vi "Command Started.vi"(8 "error in (no error)":errorcluster, 11 "Command in":refnum<class "Command.lvclass">) -> (0 "error out":errorcluster, 3 "Command out":refnum<class "Command.lvclass">)   [LabVIEW 2013, in "Robot Actors.lvlib" / "Command.lvlib" / "Command.lvclass"]
uses:
  Command.lvclass
  Command States.ctl
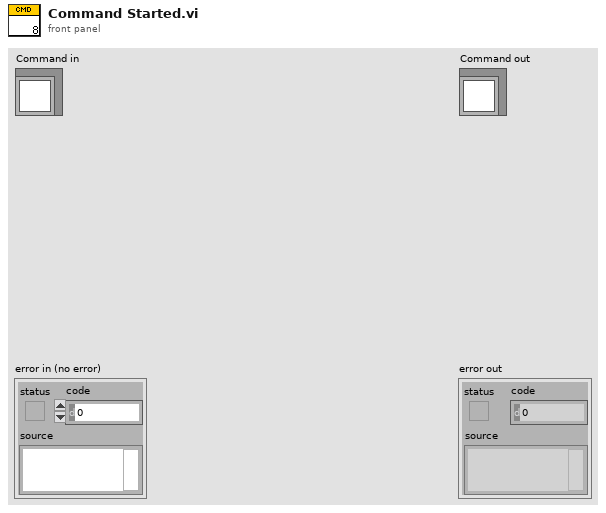
[diagram p1: front panel]
types:
  T1 = typedef "Robot Actors.lvlib/Command.lvlib/Command.lvclass/Command States.ctl" = enum16{"Unknown", "Started", "Stopped", "Finished"}
  T2 = typedef "Robot Actors.lvlib/Command.lvlib/Command.lvclass/Command Status.ctl" = cluster{"Command Name":string, "Command Start Time":timestamp, "Command End Time":timestamp, "Is Command Finished?":bool, "Command ID":dbl, "Command State":T1}
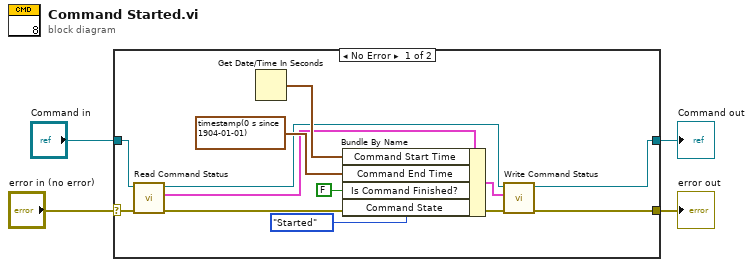
[diagram p0: block diagram]
diagram:
  n1 = case shown="No Error" "error in (no error)" {
    selector: "error in (no error)" -> [w8 w18]
    tunnel: [w6 w18] -> w3
    tunnel: [w10 w17] -> w1
    tunnel: "Command in" -> [w11 w17]
    frame No Error {
      n2 = call-dynamic "Read Command Status.vi"("error in (no error)"=w8, "Command in"=w11) -> ("error out"=w7:errorcluster, "Command Status"=w14:T2, "Command out"=w13:refnum<class "Command.lvclass">)  [unwired: 7 in]
      n3 = Get Date/Time In Seconds() -> (seconds since 1Jan1904=w15:timestamp)
      n4 = Bundle By Name(cluster=w14, "Command Start Time"=w15, "Command End Time"=timestamp(0 s since 1904-01-01), "Is Command Finished?"=FALSE, "Command State"=Command_States."Started") -> (w12:T2)
      n5 = call-dynamic "Write Command Status.vi"("error in (no error)"=w7, "Command Status"=w12, "Command in"=w13) -> ("error out"=w6:errorcluster, "Command out"=w10:refnum<class "Command.lvclass">)  [unwired: 7 in]
    }
    frame Error {
    }
  }
  "error out" <- w3
  "Command out" <- w1
